vi "RT Driver VI.vi"(6 "Device Clock":string, 9 "Device Inputs FIFO":refnum<k33>, 10 "Device Outputs FIFO":refnum<k33>, 11 "Device Reference":T1 format="%.0x") -> ()   [LabVIEW 2016, in "UDP Sender Engine.lvlib"]
uses:
  UDP Sender Engine.lvlib
  <vilib>/NI Veristand/Custom Device API/Custom Device Item Ref.ctl
  <vilib>/NI Veristand/Custom Device API/Custom Device Channel Type.ctl
  Shared/Constants.vi
  <vilib>/NI Veristand/Custom Device API/Get Item Property (String).vi
  <vilib>/NI Veristand/Custom Device API/Get Item Property (U16).vi
  <vilib>/NI Veristand/Custom Device API/Custom Device API.lvlib
  <vilib>/NI Veristand/Custom Device Tools/Custom Device Utility Library/Custom Device Utility Library.lvlib
  Shared/UDP Sender Shared.lvlib
panel:
  in  "Initialization Status Notifier":refnum<notifier>
  in  "Status Notifier":refnum<notifier>
  # "Custom Device Template\nv1.0"
  # "Use this template as a starting point for creating a custom device code module. The input controls shown here are specially named controls that the system will use to provide the device loop with data. The controls are not required for the device loop to run. For instance, if the device doesn't produce any output data, then you don't need the Device Outputs FIFO control. If you do use these controls, however, they need to have these exact names to be functional."
  # "The optional status notifier element is used to notify the RT engine of the last state of the custom device, and to indicate the device has completed execution. If this control is not used, a default No Error value is returned to the system when the device finishes execution.\n\nNote: This error state is not checked until the system shuts down. Use an output status channel to send more immediate status values to the system."
  # "This optional input can be used to send the VeriStand Engine the final status of the custom device initalization process. If this control exists on the custom device front panel, the VeriStand Engine will wait for a status update before starting up. If the custom device reports an error, that will abort the execution of the current configuration in the VeriStand Engine.\n\nThis control can be deleted if the custom device does not need to send the initialization status update."
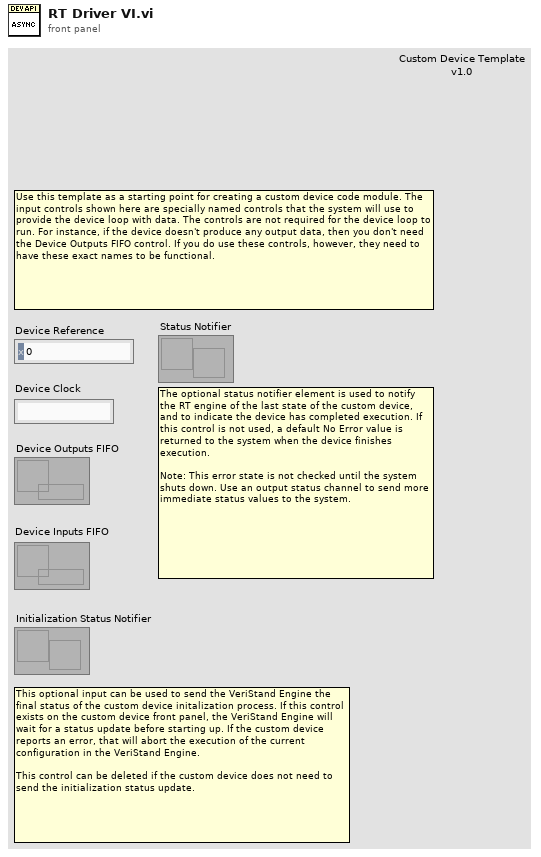
[diagram p1: front panel]
types:
  T1 = typedef "Custom Device API.lvlib/Custom Device Item Ref.ctl" = u64
  T2 = typedef "Custom Device API.lvlib/Custom Device Channel Type.ctl" = enum16{"Input", "Output"}
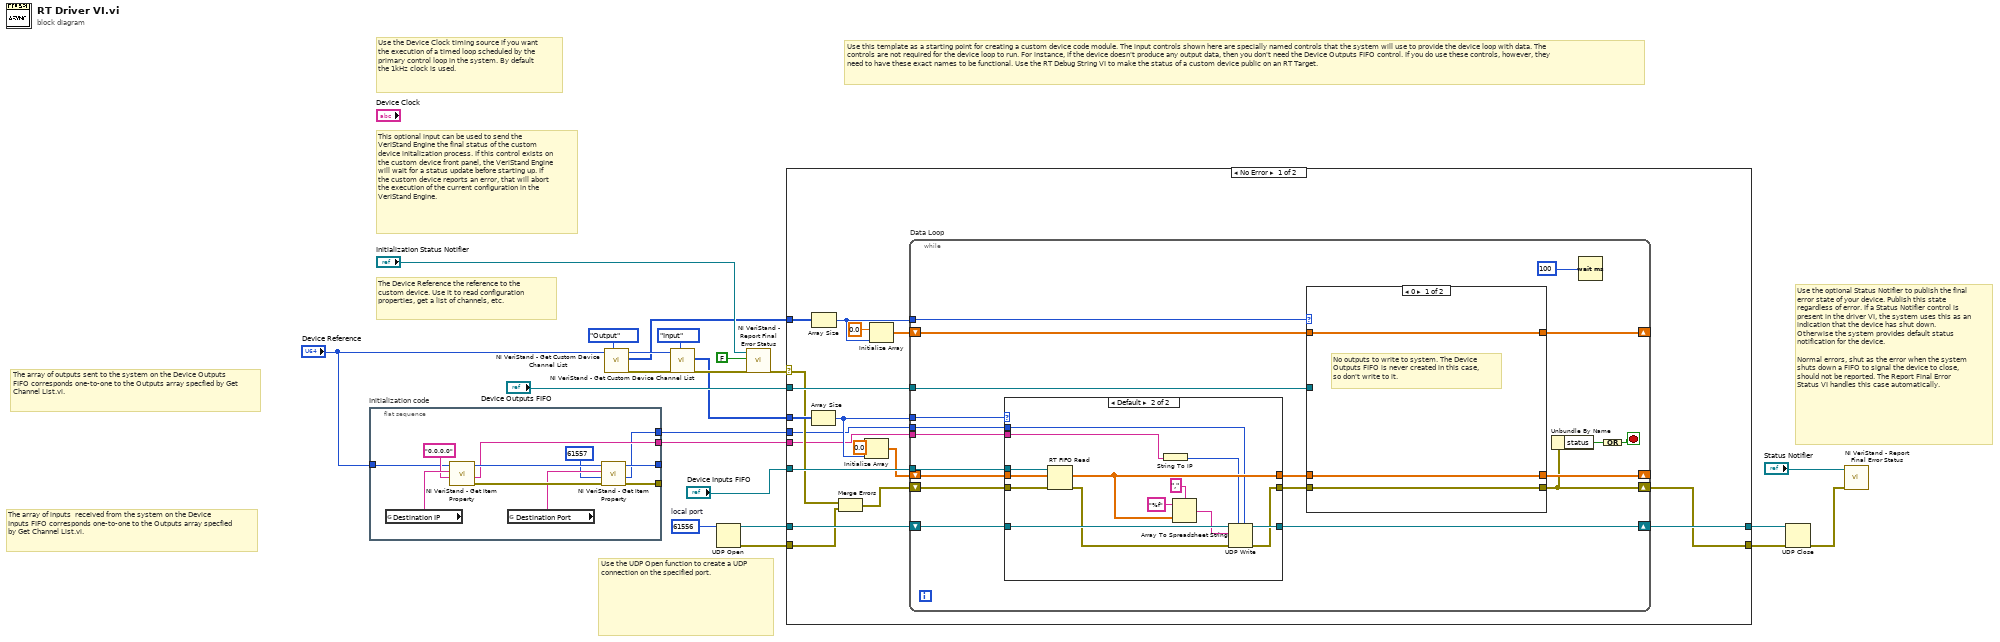
[diagram p0: block diagram]
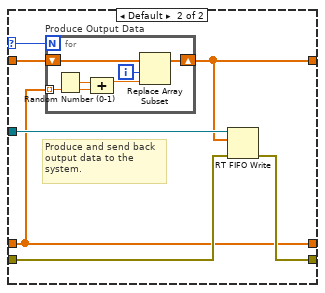
[diagram p2: hidden frame]
diagram:
  w9 = u16 61556  # local port
  # "Use the UDP Open function to create a UDP connection on the specified port."
  # "This optional input can be used to send the VeriStand Engine the final status of the custom device initalization process. If this control exists on the custom device front panel, the VeriStand Engine will wait for a status update before starting up. If the custom device reports an error, that will abort the execution of the current configuration in the VeriStand Engine."
  # "The array of inputs  received from the system on the Device Inputs FIFO corresponds one-to-one to the Outputs array specfied by Get Channel List.vi."
  # "Use the optional Status Notifier to publish the final error state of your device. Publish this state regardless of error. If a Status Notifier control is present in the driver VI, the system uses this as an indication that the device has shut down. Otherwise the system provides default status notification for the device.\n\nNormal errors, shut as the error when the system shuts down a FIFO to signal the device to close, should not be reported. The Report Final Error Status VI handles this case automatically."
  # "The array of outputs sent to the system on the Device Outputs FIFO corresponds one-to-one to the Outputs array specfied by Get Channel List.vi."
  # "The Device Reference the reference to the custom device. Use it to read configuration properties, get a list of channels, etc."
  # "Use the Device Clock timing source if you want the execution of a timed loop scheduled by the primary control loop in the system. By default the 1kHz clock is used."
  # "Use this template as a starting point for creating a custom device code module. The input controls shown here are specially named controls that the system will use to provide the device loop with data. The controls are not required for the device loop to run. For instance, if the device doesn't produce any output data, then you don't need the Device Outputs FIFO control. If you do use these controls, however, they need to have these exact names to be functional. Use the RT Debug String VI to make the status of a custom device public on an RT Target."
  n1 = flat-sequence "Initialization code" {
    tunnel: [w29] -> _
    tunnel: [w28] -> _
    tunnel: "Device Reference" -> [w25]
    tunnel: [w24] -> w2
    tunnel: [w23] -> w1
    frame #0 {
      n2 = global read "Constants.vi" "Destination IP"() -> (w33:string)
      n3 = call-poly <vilib>:"NI VeriStand - Get Item Property.vi"("Default Value"="0.0.0.0", "Property Name"=w33, "Item Ref in"=w25) -> ("error out"=w30:errorcluster, "Value"=w24:string, "Item Ref out"=w31:T1)  [unwired: 5 in, 1 out]
      n4 = global read "Constants.vi" "Destination Port"() -> (w27:string)
      n5 = call-poly <vilib>:"NI VeriStand - Get Item Property.vi"("error in (no error)"=w30, "Default Value"=u16 61557, "Property Name"=w27, "Item Ref in"=w31) -> ("error out"=w29:errorcluster, "Value"=w23:u16, "Item Ref out"=w28:T1)  [unwired: 4 in, 1 out]
    }
  }
  n6 = call <vilib>:"NI VeriStand - Get Custom Device Channel List.vi"("Channel Type"=Custom_Device_Channel_Type."Output", "Device Ref in"="Device Reference") -> ("error out"=w16:errorcluster, "Specified Channel Ref List"=w13:T1[], "Device Ref out"=w17:T1)  [unwired: 1 in, 6 out]
  n7 = call <vilib>:"NI VeriStand - Get Custom Device Channel List.vi"("Channel Type"=Custom_Device_Channel_Type."Input", "error in (no error)"=w16, "Device Ref in"=w17) -> ("error out"=w22:errorcluster, "Specified Channel Ref List"=w14:T1[])  [unwired: 7 out]
  n8 = UDP Open(11:w9) -> (port=w8:refnum<k16>, 0:w7:errorcluster)  [unwired: 4 in, 1 out]
  n9 = call <vilib>:"NI VeriStand - Report Final Error Status.vi"("error in (no error)"=w22, "Filter FIFO & Shutdown Errors (T)"=FALSE ("Filter FIFO Errors (T)"), "Status Notifier"="Initialization Status Notifier") -> ("error out"=w11:errorcluster)  [unwired: 8 out]
  n10 = case shown="No Error" w11 {
    selector: w11 -> [w40 w105]
    tunnel: "Device Outputs FIFO" -> [w51 _]
    tunnel: "Device Inputs FIFO" -> [w50 _]
    tunnel: w14 -> [w44 _]
    tunnel: w13 -> [w43 _]
    tunnel: w8 -> [w41 w104]
    tunnel: w7 -> [w39 _]
    tunnel: [w37 w104] -> w6
    tunnel: [w36 w105] -> w5
    tunnel: w2 -> [w35 _]
    tunnel: w1 -> [w34 _]
    frame No Error {
      n11 = Array Size(array=w44) -> (size(s)=w42:i32)
      n12 = Array Size(array=w43) -> (size(s)=w45:i32)
      n13 = Merge Errors(w40, w39) -> (w38:errorcluster)
      n14 = Initialize Array(0.0 ("element"), w42) -> (w46:dbl[])
      n15 = Initialize Array(0.0 ("element"), w45) -> (w47:dbl[])
      n16 = while "Data Loop" {
        shift-right: [w59] -> _
        shift-left: w46 -> [w69]
        shift-right: [w54] -> w36
        shift-left: w38 -> [w70]
        shift-right: [w67] -> _
        shift-left: w47 -> [w68]
        tunnel: w45 -> [w64]
        tunnel: w51 -> [w66]
        tunnel: w50 -> [w65]
        tunnel: w42 -> [w63]
        shift-right: [w57] -> w37
        shift-left: w41 -> [w58]
        tunnel: w35 -> [w53]
        tunnel: w34 -> [w52]
        stop <- w55 stop-if-true
        n17 = case shown="Default" w63 {
          tunnel: w65 -> [_ w103]
          tunnel: w69 -> [w89 w102]
          tunnel: [w89 w94] -> w62
          tunnel: [w88 w97] -> w61
          tunnel: w70 -> [w88 w101]
          tunnel: w58 -> [w87 w100]
          tunnel: [w87 w99] -> w57
          tunnel: w53 -> [_ w91]
          tunnel: w52 -> [_ w90]
          frame 0 {
            # "No inputs to read\nfrom system. Inputs FIFO not created in this case, so don't write to it."
          }
          frame Default {
            n18 = RT FIFO Read(0:w103, 1:w102, 3:w101) -> (9:w94:dbl[], 11:w98:errorcluster)  [unwired: 4 out]
            n19 = String To IP(1:w91) -> (0:w92:u32)
            n20 = Array To Spreadsheet String(delimiter (Tab)=",", array=w94, 3:"%f" ("format string")) -> (spreadsheet string=w93:string)
            n21 = UDP Write(address=w92, port or service name=w90, connection ID=w100, data in=w93, 8:w98) -> (error out=w97:errorcluster, 3:w99:refnum<k16>)  [unwired: 1 in]
          }
        }
        n22 = case shown="0" w64 {
          selector: w64 -> [_ w74]
          tunnel: w66 -> [_ w80]
          tunnel: w68 -> [w73 w79]
          tunnel: w62 -> [w72 w75]
          tunnel: w61 -> [w71 w78]
          tunnel: [w71 w77] -> w54
          tunnel: [w73 w76] -> w67
          tunnel: [w72 w75] -> w59
          frame 0 {
            # "No outputs to write to system. The Device Outputs FIFO is never created in this case, so don't write to it."
          }
          frame Default {
            # "Produce and send back output data to the system."
            n23 = for "Produce Output Data" {
              N: w74 -> [_]
              shift-right: [w85] -> w76
              shift-left: w79 -> [w86]
              tunnel: w75 -> [w81] mode=indexing
              i -> [w84]
              n24 = Random Number (0-1)() -> (number: 0 to 1=w83:dbl)
              n25 = Compound Arithmetic op=ADD(w83, w81) -> (w82:dbl)
              n26 = Replace Array Subset(array=w86, new element=w82, index=w84) -> (w85:dbl[])
            }
            n27 = RT FIFO Write(0:w80, 1:w76, 3:w78) -> (11:w77:errorcluster)  [unwired: 1 in, 4 out]
          }
        }
        n28 = Unbundle By Name(w54) -> ("status"=w56:bool)
        n29 = Wait (ms)(milliseconds to wait=u32 100) -> ()  [unwired: 1 out]
        n30 = Compound Arithmetic op=OR(w56) -> (w55:bool)
      }
    }
    frame Error {
    }
  }
  n31 = UDP Close(connection ID=w6, 8:w5) -> (error out=w4:errorcluster)  [unwired: 1 out]
  n32 = call <vilib>:"NI VeriStand - Report Final Error Status.vi"("error in (no error)"=w4, "Status Notifier"="Status Notifier") -> ()  [unwired: 1 in, 9 out]
